vi "Pot Point.vi"(7 "Encapsulant":string, 8 "error in (no error)":errorcluster, 10 "Point":refnum<class "Vec3d.lvclass">, 11 "Gantry in":refnum<class "Gantry.lvclass">) -> (0 "error out":errorcluster, 3 "Gantry out":refnum<class "Gantry.lvclass">)   [LabVIEW 2017, in "Gantry.lvclass"]
uses:
  Gantry.lvclass
  Vec3d Class/Vec3d.lvclass
  FlexWorktable/FlexWorktable.lvclass
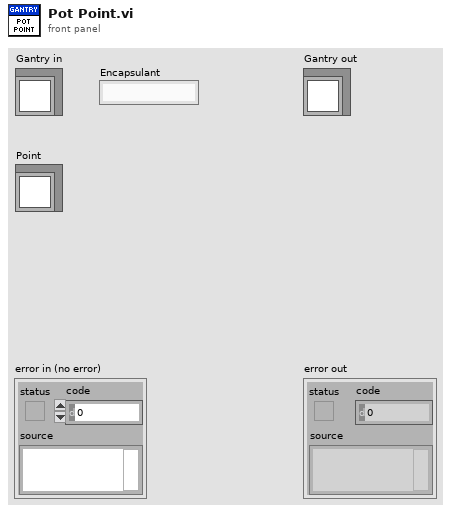
[diagram p1: front panel]
types:
  T1 = cluster{"Syringe Holder":string, "Mixing Time":timestamp, "Tip Offset":refnum<class "Vec3d.lvclass">}
  T2 = typedef "FlexWorktable.lvclass/Potting Parameters.ctl" = cluster{"Curing Param A":dbl, "Curing Param B":dbl, "Speed Nominal":dbl, "Time Nominal":dbl, "Turn-on Time":dbl, "Turn-off Time":dbl, "Safe Height Offset":dbl, "Tip Height":dbl}
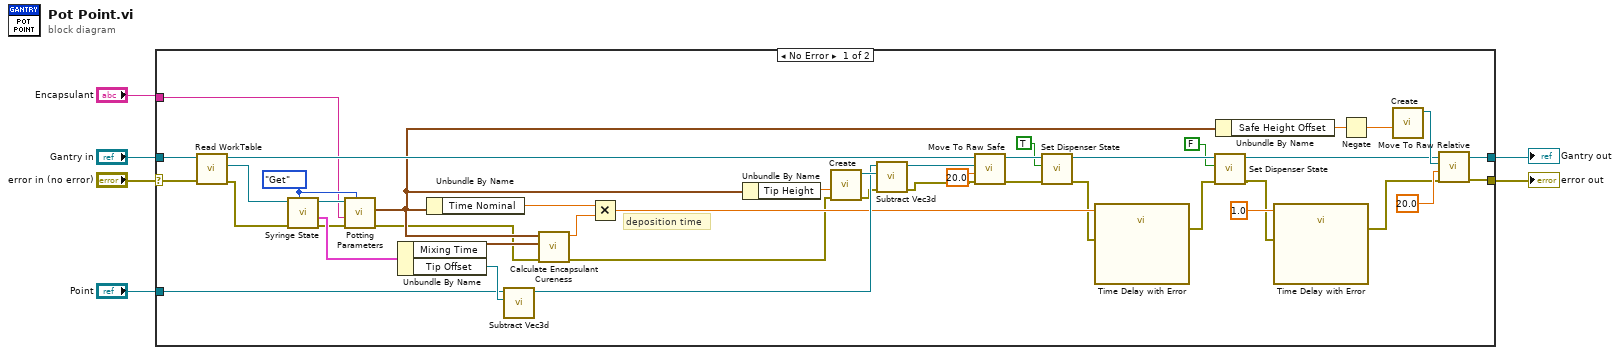
[diagram p0: block diagram]
diagram:
  n1 = case shown="No Error" "error in (no error)" {
    selector: "error in (no error)" -> [w20 w51]
    tunnel: [w48 w51] -> w1
    tunnel: [w49 w50] -> w2
    tunnel: "Gantry in" -> [w21 w50]
    tunnel: "Point" -> [w35 _]
    tunnel: "Encapsulant" -> [w15 _]
    frame No Error {
      w16 = enum16{"Get", "Set"}."Get" ("Get/Set")
      # "deposition time"
      n2 = call-dynamic "Read WorkTable.vi"("error in"=w20, "Gantry Class in"=w21) -> ("error out"=w19:errorcluster, "Worktable"=w23:refnum<class "FlexWorktable.lvclass">, "Gantry Class out"=w47:refnum<class "Gantry.lvclass">)  [unwired: 7 in]
      n3 = call-dynamic "Syringe State.vi"("Get/Set"=w16, "error in (no error)"=w19, "FlexWorktable in"=w23) -> ("error out"=w17:errorcluster, "Syringe out"=w22:T1, "FlexWorktable out"=w18:refnum<class "FlexWorktable.lvclass">)  [unwired: 6 in]
      n4 = call-dynamic "Potting Parameters.vi"("Get/Set"=w16, "error in (no error)"=w17, "Encapsulant"=w15, "FlexWorktable in"=w18) -> ("error out"=w10:errorcluster, "Potting Parameters out"=w11:T2)  [unwired: 5 in, 1 out]
      n5 = Unbundle By Name(w22) -> ("Mixing Time"=w37:timestamp, "Tip Offset"=w46:refnum<class "Vec3d.lvclass">)
      n6 = Unbundle By Name(w11) -> ("Time Nominal"=w12:dbl)
      n7 = call "Subtract Vec3d.vi"("Vec3d in 2"=w46, "Vec3d in 1"=w35) -> ("Vec3d Class out"=w34:refnum<class "Vec3d.lvclass">)  [unwired: 8 in, 1 out]
      n8 = call "Calculate Encapsulant Cureness.vi"("error in"=w10, "Mixing Time"=w37, "Potting Parameters"=w11) -> ("error out"=w9:errorcluster, "Cureness"=w36:dbl)  [unwired: 7 in]
      n9 = Multiply(x=w12, y=w36) -> (x*y=w26:dbl)
      n10 = Unbundle By Name(w11) -> ("Tip Height"=w14:dbl)
      n11 = call "Create.vi"("error in"=w9, "Z"=w14) -> ("error out"=w32:errorcluster, "Vec3d Class out"=w38:refnum<class "Vec3d.lvclass">)  [unwired: 8 in]
      n12 = call "Subtract Vec3d.vi"("error in (no error)"=w32, "Vec3d in 2"=w38, "Vec3d in 1"=w34) -> ("error out"=w31:errorcluster, "Vec3d Class out"=w39:refnum<class "Vec3d.lvclass">)  [unwired: 7 in]
      n13 = call-dynamic "Move To Raw Safe.vi"("error in"=w31, "Speed(mm/s)"=20.0, "Destination"=w39, "Gantry in"=w47) -> ("error out"=w45:errorcluster, "Gantry out"=w44:refnum<class "Gantry.lvclass">)  [unwired: 6 in]
      n14 = call-dynamic "Set Dispenser State.vi"("error in"=w45, "On/Off"=TRUE, "Gantry in"=w44) -> ("error out"=w25:errorcluster, "Gantry out"=w33:refnum<class "Gantry.lvclass">)  [unwired: 7 in]
      n15 = call "Time Delay with Error.vi"("error in (no error)"=w25, "Delay Time (s)"=w26) -> ("error out"=w24:errorcluster)  [unwired: 9 in]
      n16 = call-dynamic "Set Dispenser State.vi"("error in"=w24, "On/Off"=FALSE, "Gantry in"=w33) -> ("error out"=w28:errorcluster, "Gantry out"=w30:refnum<class "Gantry.lvclass">)  [unwired: 7 in]
      n17 = Unbundle By Name(w11) -> ("Safe Height Offset"=w13:dbl)
      n18 = call "Time Delay with Error.vi"("error in (no error)"=w28, "Delay Time (s)"=1.0) -> ("error out"=w27:errorcluster)  [unwired: 9 in]
      n19 = Negate(x=w13) -> (-x=w42:dbl)
      n20 = call "Create.vi"("Z"=w42) -> ("Vec3d Class out"=w43:refnum<class "Vec3d.lvclass">)  [unwired: 9 in, 1 out]
      n21 = call-dynamic "Move To Raw Relative.vi"("error in"=w27, "Speed(mm/s)"=20.0, "Delta"=w43, "Gantry in"=w30) -> ("error out"=w48:errorcluster, "Gantry out"=w49:refnum<class "Gantry.lvclass">)  [unwired: 6 in]
    }
    frame Error {
    }
  }
  "error out" <- w1
  "Gantry out" <- w2
